vi "手控.vi"() -> ()   [LabVIEW 2018]
panel:
  in  "右":dbl
  in  "オ":dbl
  in  "stop":bool
  out "手控轉速":dbl
  out "轉速差手控":dbl
  out "appended array":bool[](array[boolean])
  in  "手控":T1 {"手控轉速" scale=0.0..3000.0; "轉速差手控" scale=0.0..2000.0}
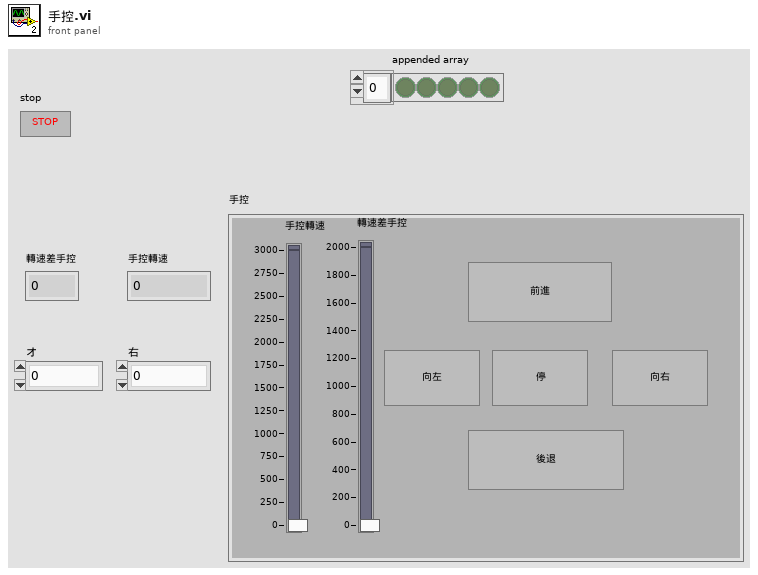
[diagram p1: front panel]
types:
  T1 = cluster{"轉速差手控":dbl, "手控轉速":dbl, "前進":bool, "向左":bool, "向右":bool, "後退":bool, "停":bool}
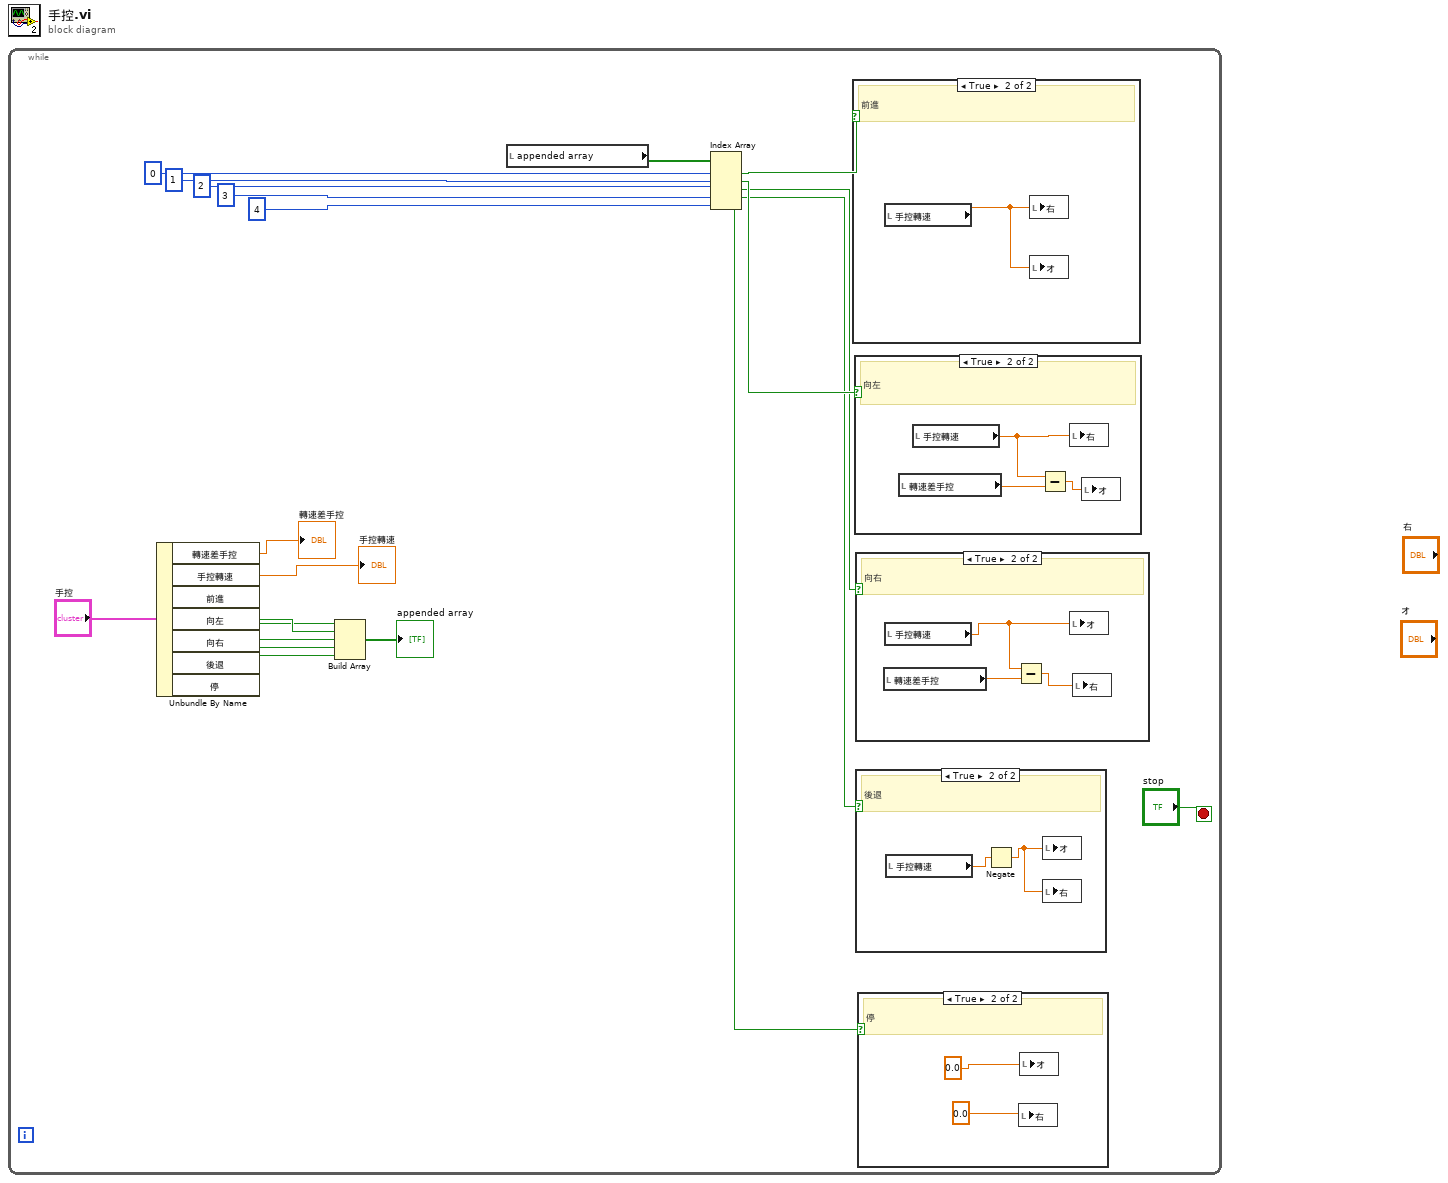
[diagram p0: block diagram]
diagram:
  n1 = while {
    stop <- "stop" stop-if-true
    n2 = Unbundle By Name("手控") -> ("轉速差手控"=→"轉速差手控":dbl, "手控轉速"=→"手控轉速":dbl, "前進"=w14:bool, "向左"=w15:bool, "向右"=w16:bool, "後退"=w17:bool, "停"=w18:bool)
    n3 = Build Array(w14, w15, w16, w17, w18) -> (→"appended array":bool[])
    n4 = local read "appended array"() -> (w11:bool[])
    n5 = Index Array(array=w11, index #1=0 ("index"), index #2=1 ("index"), index #3=2 ("index"), index #4=3 ("index"), index #5=4 ("index")) -> (element #1=w12:bool, element #2=w4:bool, element #3=w3:bool, element #4=w2:bool, element #5=w1:bool)
    n6 = case shown="True" w12 {
      frame False {
      }
      frame True {
        # "前進"
        n7 = local read "手控轉速"() -> (w32:dbl)
        n8 = local write "右"(w32) -> ()
        n9 = local write "オ"(w32) -> ()
      }
    }
    n10 = case shown="True" w4 {
      frame False {
      }
      frame True {
        # "向左"
        n11 = local read "轉速差手控"() -> (w30:dbl)
        n12 = local read "手控轉速"() -> (w31:dbl)
        n13 = Subtract(x=w31, y=w30) -> (x-y=w29:dbl)
        n14 = local write "右"(w31) -> ()
        n15 = local write "オ"(w29) -> ()
      }
    }
    n16 = case shown="True" w3 {
      frame False {
      }
      frame True {
        # "向右"
        n17 = local read "轉速差手控"() -> (w26:dbl)
        n18 = local read "手控轉速"() -> (w28:dbl)
        n19 = Subtract(x=w28, y=w26) -> (x-y=w27:dbl)
        n20 = local write "オ"(w28) -> ()
        n21 = local write "右"(w27) -> ()
      }
    }
    n22 = case shown="True" w2 {
      frame False {
      }
      frame True {
        # "後退"
        n23 = local read "手控轉速"() -> (w25:dbl)
        n24 = Negate(x=w25) -> (-x=w24:dbl)
        n25 = local write "オ"(w24) -> ()
        n26 = local write "右"(w24) -> ()
      }
    }
    n27 = case shown="True" w1 {
      frame False {
      }
      frame True {
        # "停"
        n28 = local write "右"(0.0) -> ()
        n29 = local write "オ"(0.0) -> ()
      }
    }
  }
